vi "US300 Depth Sensor Driver Scan Interface.vi"() -> ()   [LabVIEW 2011]
panel:
  in  "stop":bool
  out "Waveform Chart":dbl(graph)
  out "error out":errorcluster
  in  "Wait ms":dbl
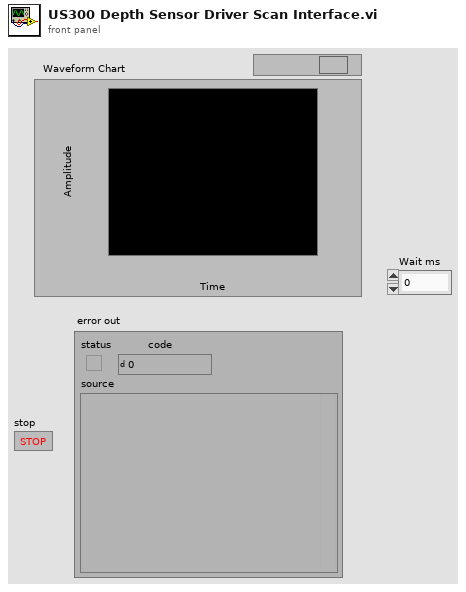
[diagram p1: front panel]
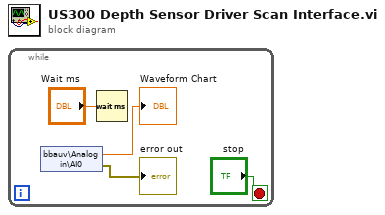
[diagram p0: block diagram]
diagram:
  n1 = while {
    stop <- "stop" stop-if-true
    n2 = shared-variable "bbauv\\Analog in\\AI0"() -> (→"Waveform Chart":dbl, error out=→"error out":errorcluster)  [unwired: 1 in]
    n3 = Wait (ms)(milliseconds to wait="Wait ms") -> ()  [unwired: 1 out]
  }
